vi "createReaderQueue.vi"(0 "QueueName":string, 5 "error in":errorcluster, 8 "ReaderEndPointName":string) -> (19 "error out":errorcluster)   [LabVIEW 2013]
doc: "Used as a mechanism to have queue notification across process boundaries using network streams. No need to define a shared variable. Put the vi outside of the loop in parallel, and define a named queue to communicate through the link.\n\nQueueName - Named queue to be used within the process.\nRemoteEndPointName - Specify to the remote TX end point where you want to push data from."
uses:
  control/payloadData.ctl
  control/cmdQueueReaderRef.ctl
  Global/GlobalStop.vi
  <resource>/objmgr/ni.dex.rc
panel:
  out "Main Loop":i32
  out "Application:Name":string
  out "Error Loop":i32
  out "Acquire loop":i32
  out "readerURL":string
  out "streamOP":T1
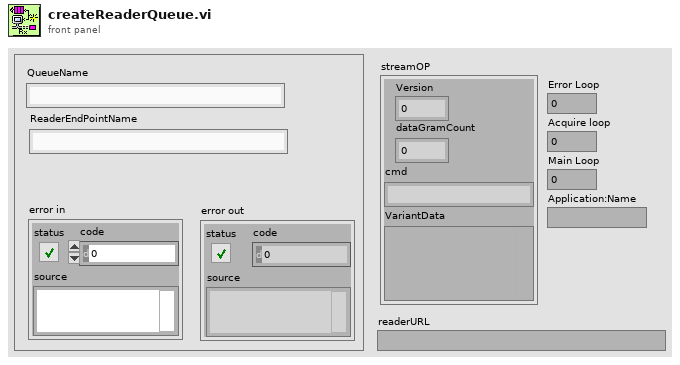
[diagram p1: front panel]
types:
  T1 = typedef "payloadData.ctl" = cluster{"Version":u32, "dataGramCount":i32, "cmd":string, "VariantData":variant}
  T2 = enum32{"invalid app kind", "Development System", "Run Time System", "Student Edition", "Embedded LabVIEW", "Evaluation", "Custom"}
  T3 = typedef "cmdQueueReaderRef.ctl" = cluster{"cmd":string, "msgQueue":refnum<queue>, "readerEndPoint":refnum<k21>}
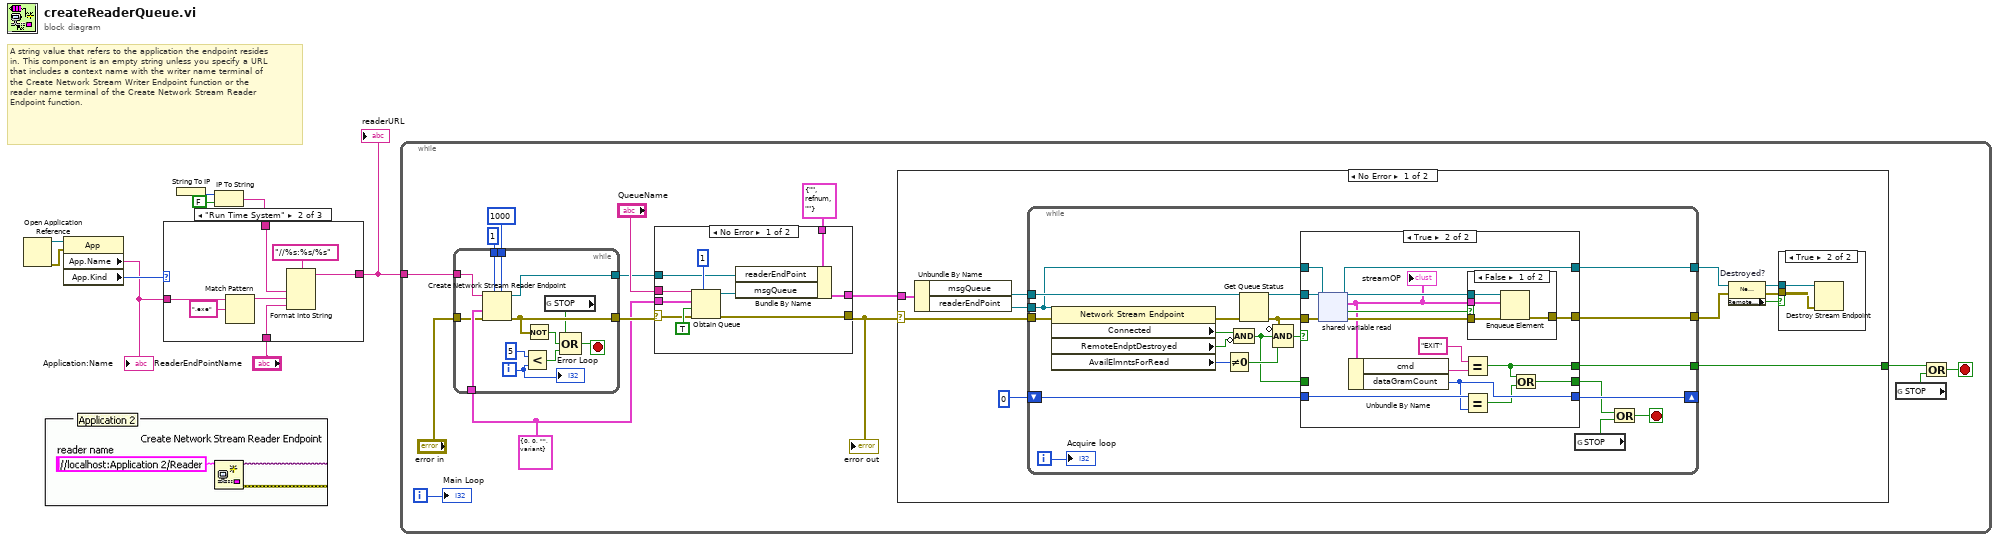
[diagram p0: block diagram]
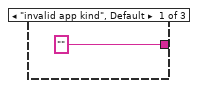
[diagram p2: hidden frame]
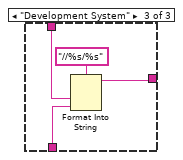
[diagram p3: hidden frame]
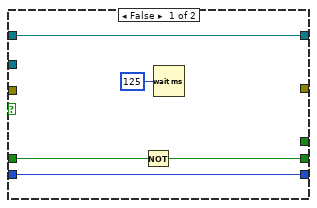
[diagram p5: hidden frame]
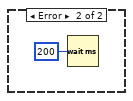
[diagram p7: hidden frame]
diagram:
  # "A string value that refers to the application the endpoint resides in. This component is an empty string unless you specify a URL that includes a context name with the writer name terminal of the Create Network Stream Writer Endpoint function or the reader name terminal of the Create Network Stream Reader Endpoint function."
  n1 = Open Application Reference() -> (0:w8:errorcluster, 3:w9:refnum<vi>)  [unwired: 4 in]
  n2 = property class="App"(reference=w9, error in=w8) -> ("App.Name"=w2:string, "App.Kind"=w3:T2)  [unwired: 2 out]
  "Application:Name" <- w2
  n3 = String To IP() -> (0:w6:u32)  [unwired: 1 in]
  n4 = IP To String(1:FALSE ("dot notation? (F)"), 2:w6) -> (0:w4:string)
  n5 = case shown="\"Run Time System\"" w3 {
    tunnel: ["" w16 w20] -> w1
    tunnel: "ReaderEndPointName" -> [_ w15 w18]
    tunnel: w4 -> [_ w14 w19]
    tunnel: w2 -> [_ w13 _]
    frame "invalid app kind", Default {
    }
    frame "Run Time System" {
      n6 = Match Pattern(string=w13, regular expression=".exe") -> (before substring=w11:string)  [unwired: 1 in, 3 out]
      n7 = Format Into String(format string="//%s:%s/%s", w14, w11, w15) -> (resulting string=w16:string)  [unwired: 2 in, 1 out]
    }
    frame "Development System" {
      n8 = Format Into String(format string="//%s/%s", w19, w18) -> (resulting string=w20:string)  [unwired: 2 in, 1 out]
    }
  }
  "readerURL" <- w1
  n9 = while {
    tunnel: w1 -> [w26]
    i -> [w25]
    stop <- w22 stop-if-true
    w34 = T1 {"Version"=0, "dataGramCount"=0, "cmd"="", "VariantData"=variant} ("Data")
    n10 = while {
      tunnel: w34 -> [w109]
      tunnel: [w108] -> w33
      tunnel: "error in" -> [w107]
      tunnel: [w104] -> w36
      tunnel: 1000 ("timeout in ms (-1)") -> [w100]
      tunnel: 1 ("writer buffer size") -> [w99]
      tunnel: w26 -> [w98]
      i -> [w106]
      stop <- w101 stop-if-true
      n11 = Create Network Stream Reader Endpoint(5:w100, 7:w99, 8:w107, 9:w109, 11:w98) -> (0:w104:errorcluster, 3:w108:refnum<k21>)  [unwired: 2 in]
      n12 = Less?(x=5, y=w106) -> (x < y?=w103:bool)
      n13 = Not(x=w104) -> (.not. x?=w102:bool)
      n14 = global read "GlobalStop.vi" "STOP"() -> (w97:bool)
      n15 = Compound Arithmetic op=OR(w97, w102, w103) -> (w101:bool)
      "Error Loop" <- w106
    }
    n16 = case shown="No Error" w36 {
      selector: w36 -> [w115 w120]
      tunnel: [w119 _] -> w30
      tunnel: [w118 w120] -> w29
      tunnel: "QueueName" -> [w117 _]
      tunnel: w34 -> [w114 _]
      tunnel: w33 -> [w111 _]
      tunnel: T3 {"cmd"="", "msgQueue"=refnum, "readerEndPoint"=""} ("msgRef") -> [w110 _]
      frame No Error {
        n17 = Obtain Queue(max queue size (-1, unlimited)=1 ("writer buffer size"), name (unnamed)=w117, element data type=w114, create if not found? (T)=TRUE, error in (no error)=w115) -> (queue out=w113:refnum<queue>, error out=w118:errorcluster)  [unwired: 1 out]
        n18 = Bundle By Name(cluster=w110, "readerEndPoint"=w111, "msgQueue"=w113) -> (w119:T3)
      }
      frame Error {
      }
    }
    "error out" <- w29
    n19 = case shown="No Error" w29 {
      selector: w29 -> [w45 _]
      tunnel: w30 -> [w47 _]
      tunnel: [w42 _] -> w24
      frame No Error {
        n20 = Unbundle By Name(w47) -> ("msgQueue"=w44:refnum<queue>, "readerEndPoint"=w46:refnum<k21>)
        n21 = while {
          tunnel: w46 -> [w62]
          tunnel: w45 -> [w70]
          tunnel: w44 -> [w69]
          shift-right: [w58] -> _
          shift-left: 0 -> [w59]
          tunnel: [w57] -> w42
          tunnel: [w56] -> w38
          tunnel: [w55] -> w37
          i -> [w54]
          stop <- w51 stop-if-true
          n22 = property class="Network Stream Endpoint"(reference=w62, error in=w70) -> (error out=w65:errorcluster, "Connected"=w68:bool, "RemoteEndptDestroyed"=w67:bool, "AvailElmntsForRead"=w66:i32)  [unwired: 1 out]
          n23 = Not Equal To 0?(x=w66) -> (x != 0?=w64:bool)
          n24 = Compound Arithmetic op=AND(w68, invert w67) -> (w53:bool)
          n25 = Get Queue Status(queue=w69, error in (no error)=w65) -> (queue out=w60:refnum<queue>, error out=w61:errorcluster)  [unwired: 1 in, 6 out]
          n26 = Compound Arithmetic op=AND(invert w61, w53, w64) -> (w63:bool)
          n27 = case shown="True" w63 {
            tunnel: w62 -> [w73 w90]
            tunnel: w61 -> [_ w89]
            tunnel: w60 -> [_ w88]
            tunnel: w59 -> [w74 w82]
            tunnel: [w74 w81] -> w58
            tunnel: [w71 w79] -> w52
            tunnel: [_ w78] -> w57
            tunnel: [w73 w77] -> w56
            tunnel: [_ w76] -> w55
            tunnel: w53 -> [w72 _]
            frame False {
              n28 = Not(x=w72) -> (.not. x?=w71:bool)
              n29 = Wait (ms)(milliseconds to wait=u32 125) -> ()  [unwired: 1 out]
            }
            frame True {
              n30 = shared-variable-read(w90, w89) -> (w77:refnum<k21>, w87:errorcluster, w86:bool, w85:T1)  [unwired: 1 in]
              "streamOP" <- w85
              n31 = Unbundle By Name(w85) -> ("cmd"=w84:string, "dataGramCount"=w81:i32)
              n32 = Equal?(x="EXIT", y=w84) -> (x = y?=w78:bool)
              n33 = Equal?(x=w82, y=w81) -> (x = y?=w80:bool)
              n34 = case shown="False" w86 {
                tunnel: w88 -> [w94 _]
                tunnel: w87 -> [w93 w95]
                tunnel: w85 -> [w92 _]
                tunnel: [w91 w95] -> w76
                frame False {
                  n35 = Enqueue Element(queue=w94, element=w92, error in (no error)=w93) -> (error out=w91:errorcluster)  [unwired: 1 in, 2 out]
                }
                frame True {
                }
              }
              n36 = Or(x=w78, y=w80) -> (x .or. y?=w79:bool)
            }
          }
          n37 = global read "GlobalStop.vi" "STOP"() -> (w50:bool)
          n38 = Or(x=w52, y=w50) -> (x .or. y?=w51:bool)
          "Acquire loop" <- w54
        }
        n39 = property on="Destroyed?" class="Network Stream Endpoint"(reference=w38, error in=w37) -> (reference out=w40:refnum<k21>, error out=w41:errorcluster, "RemoteEndptDestroyed"=w39:bool)
        n40 = case shown="True" w39 {
          tunnel: w41 -> [_ w49]
          tunnel: w40 -> [_ w48]
          frame False {
          }
          frame True {
            n41 = Destroy Stream Endpoint(8:w49, 11:w48) -> ()  [unwired: 1 out]
          }
        }
      }
      frame Error {
        n42 = Wait (ms)(milliseconds to wait=u32 200) -> ()  [unwired: 1 out]
      }
    }
    n43 = global read "GlobalStop.vi" "STOP"() -> (w23:bool)
    n44 = Or(x=w24, y=w23) -> (x .or. y?=w22:bool)
    "Main Loop" <- w25
  }
